vi "OAT Extract Order Waveforms.vi"   [LabVIEW 2017, in "SoundVib_Gabor.lvlib"]
doc: "Extracts order waveforms from specified orders in the <B>scaled signal [EU]</B>. This VI can return order waveforms of a single order or combined orders. Use <B>orders to extract</B> to specify the desired orders. This VI does not maintain state internally; you can use this VI in a loop to process multiple blocks. Wire data to the <B>scaled signal [EU]</B> input to determine the polymorphic instance to use or manually select the instance."
uses:
  <vilib>/addons/Sound and Vibration/Order Analysis/Gabor Order Tracking/SoundVib_Gabor.lvlib
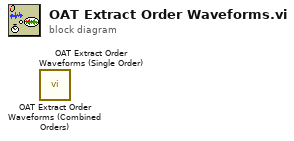
[diagram p0: block diagram]
diagram:
  n1 = call <vilib>:"OAT Extract Order Waveforms (Combined Orders).vi"() -> ()  [unwired: 11 in, 5 out]
  n2 = call <vilib>:"OAT Extract Order Waveforms (Single Order).vi"() -> ()  [unwired: 12 in, 4 out]
